vi "S2C_VLFT10_Proc_GetVersionInfo.vi"(8 "Error In":errorcluster, 11 "Item":string) -> (0 "Error Out":errorcluster, 2 "Found?":bool, 3 "Value":string)   [LabVIEW 2015]
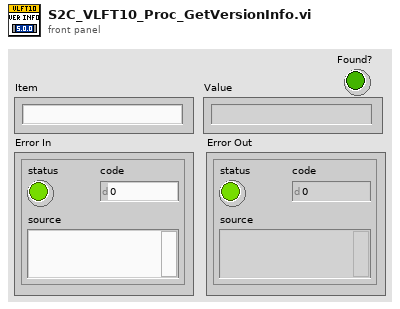
[diagram p1: front panel]
types:
  T1 = cluster{"Detected":cluster{"Items":cluster{"Name":string, "Version":string, "SubItems":cluster{"Name":string, "Version":string}[]}[], "Chassis":string}, "M_IsConsistent":bool, "Expected":string}
  T2 = cluster{"Partition":string, "Message":string, "M_ChassisSerialNumber":string, "M_SystemVersion":string, "M_Embodiment":string, "M_LastUpdateDatetime":string, "M_IsConsistent":bool, "M_NeedsConfirmation":bool, "M_ConfigurationData":string}
  T3 = cluster{"Name":string, "Version":string, "SubItems":cluster{"Name":string, "Version":string}[]}[]
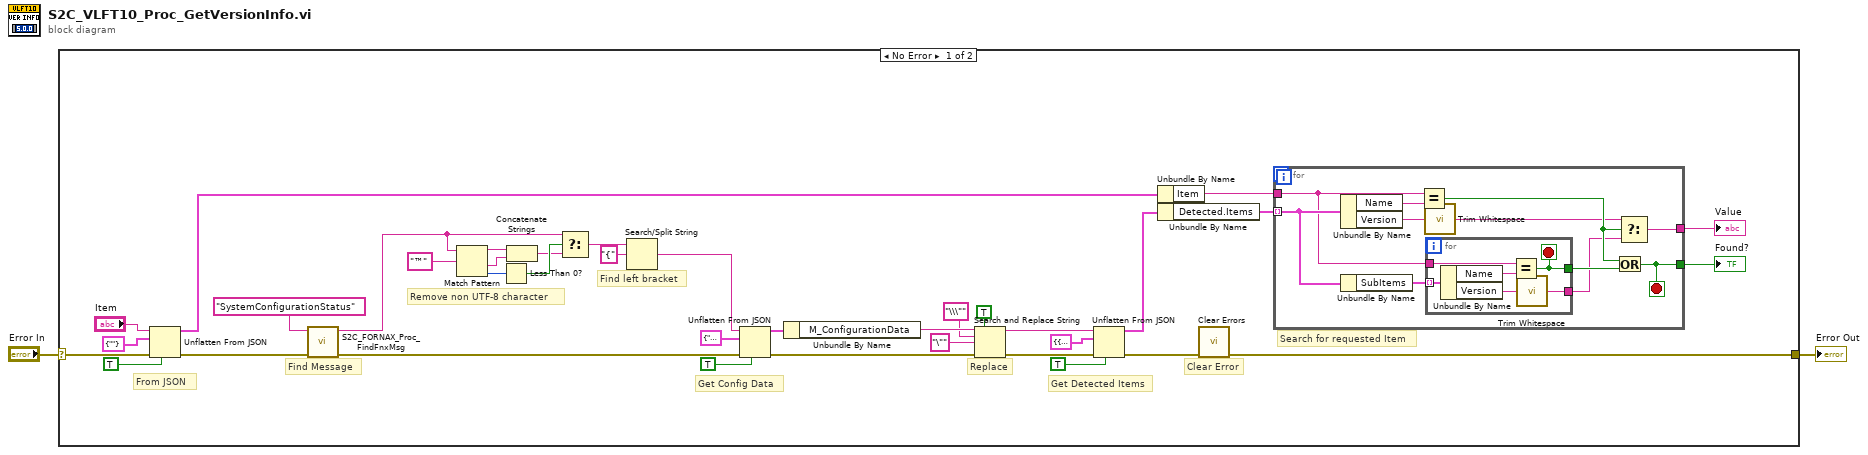
[diagram p0: block diagram]
diagram:
  n1 = case shown="No Error" "Error In" {
    selector: "Error In" -> [w22 w56]
    tunnel: [w12 w56] -> w1
    frame No Error {
      # "From JSON"
      # "Clear Error"
      # "Replace"
      # "Find Message"
      # "Search for requested Item"
      # "Find left bracket"
      # "Remove non UTF-8 character"
      # "Get Detected Items"
      # "Get Config Data"
      n2 = Unflatten From JSON(JSON string="Item", type and defaults=cluster{"Item":string} {"Item"=""}, default null elements? (F)=TRUE) -> (value=w4:cluster{"Item":string})  [unwired: 4 in, 1 out]
      n3 = call "S2C_FORNAX_Proc_FindFnxMsg.vi"("Error In"=w22, "MsgName"="SystemConfigurationStatus") -> ("Error Out"=w21:errorcluster, "Message"=w19:string)  [unwired: 8 in]
      n4 = Match Pattern(string=w19, regular expression="™") -> (before substring=w35:string, after substring=w34:string, offset past match=w33:i32)  [unwired: 1 in, 1 out]
      n5 = Less Than 0?(x=w33) -> (x < 0?=w32:bool)
      n6 = Concatenate Strings(w35, w34) -> (w31:string)
      n7 = Select(t=w19, s=w32, f=w31) -> (s? t:f=w28:string)
      n8 = Search/Split String(string=w28, search string/char (-)="{") -> (match + rest of string=w25:string)  [unwired: 1 in, 2 out]
      n9 = Unflatten From JSON(JSON string=w25, type and defaults=T2 {"Partition"="", "Message"="", "M_ChassisSerialNumber"="", "M_SystemVersion"="", "M_Embodiment"="", "M_LastUpdateDatetime"="", "M_IsConsistent"=FALSE, "M_NeedsConfirmation"=FALSE, "M_ConfigurationData"=""}, default null elements? (F)=TRUE, error in (no error)=w21) -> (value=w38:T2, error out=w16:errorcluster)  [unwired: 3 in]
      n10 = Unbundle By Name(w38) -> ("M_ConfigurationData"=w17:string)
      n11 = Search and Replace String(replace all?=TRUE ("replace all? (F)"), input string=w17, search string="\\\"", replace string="\"" ("replace string (\"\")"), error in=w16) -> (result string=w14:string, error out=w15:errorcluster)  [unwired: 3 in, 2 out]
      n12 = Unflatten From JSON(JSON string=w14, type and defaults=T1 {"Detected"={"Items"=[], "Chassis"=""}, "M_IsConsistent"=FALSE, "Expected"=""}, default null elements? (F)=TRUE, error in (no error)=w15) -> (value=w26:T1, error out=w24:errorcluster)  [unwired: 3 in]
      n13 = Unbundle By Name(w4) -> ("Item"=w3:string)
      n14 = Unbundle By Name(w26) -> ("Detected.Items"=w27:T3)
      n15 = call <vilib>:"Clear Errors.vi"("error in (no error)"=w24) -> ("error out"=w12:errorcluster)  [unwired: 5 in, 1 out]
      n16 = for {
        tunnel: w27 -> [w47] mode=indexing
        tunnel: w3 -> [w39]
        tunnel: [w41] -> w23
        tunnel: [w40] -> w13
        stop <- w40 stop-if-true
        n17 = Unbundle By Name(w47) -> ("Name"=w49:string, "Version"=w48:string)
        n18 = Unbundle By Name(w47) -> ("SubItems"=w46:cluster{"Name":string, "Version":string}[])
        n19 = Equal?(x=w39, y=w49) -> (x = y?=w44:bool)
        n20 = call <vilib>:"Trim Whitespace.vi"("string"=w48) -> ("trimmed string"=w43:string)  [unwired: 1 in]
        n21 = for {
          tunnel: w46 -> [w55] mode=indexing
          tunnel: w39 -> [w53]
          tunnel: [w50] -> w45
          tunnel: [w51] -> w42
          stop <- w50 stop-if-true
          n22 = Unbundle By Name(w55) -> ("Name"=w54:string, "Version"=w52:string)
          n23 = Equal?(x=w53, y=w54) -> (x = y?=w50:bool)
          n24 = call <vilib>:"Trim Whitespace.vi"("string"=w52) -> ("trimmed string"=w51:string)  [unwired: 1 in]
        }
        n25 = Or(x=w44, y=w45) -> (x .or. y?=w40:bool)
        n26 = Select(t=w43, s=w44, f=w42) -> (s? t:f=w41:string)
      }
      "Value" <- w23
      "Found?" <- w13
    }
    frame Error {
    }
  }
  "Error Out" <- w1
